vi "VI Tree.vi"   [LabVIEW 2018, in "TCPServer.lvlib"]
uses:
  TCPServer.lvlib
  TypeDefs/Sec Hdr CMD.ctl
  TypeDefs/Sec Hdr TLM.ctl
  TypeDefs/Connection.ctl
  TypeDefs/App.ctl
  TypeDefs/CCSDS.ctl
  fd051608-15b4-44f6-a0b0-4995f7a393de.vi
types:
  T1 = typedef "TCPServer.lvlib/Connection.ctl" = cluster{"Tcp":refnum<k5>, "Server Port":u16, "Server Port Type":enum8{"CMD", "TLM", "BOTH"}, "Client IP":string, "Client Port":u16}
  T2 = typedef "TCPServer.lvlib/CCSDS.ctl" = cluster{"Version":u8, "Type":enum8{"TLM", "CMD"}, "SecHdrFlag":bool, "AppID":u16, "SeqFlags":u8, "SeqCount":u16, "PktLength":u16}
  T3 = typedef "TCPServer.lvlib/App.ctl" = cluster{"Stack":refnum<queue>, "Cmd":cluster{"Conn":refnum<data-value>, "Daemon":refnum<vi>, "Counter":refnum<data-value>}, "Tlm":cluster{"Conn":refnum<data-value>, "Daemon":refnum<vi>, "Counter":refnum<data-value>}}
  T4 = typedef "TCPServer.lvlib/Sec Hdr TLM.ctl" = cluster{"DAYS_SINCE_2000":u16, "SECONDS_SINCE_START":u32, "MS_SINCE_START":u16}
  T5 = typedef "TCPServer.lvlib/Sec Hdr CMD.ctl" = cluster{"CMD_ID":u8, "CMD_CHECKSUM":u8}
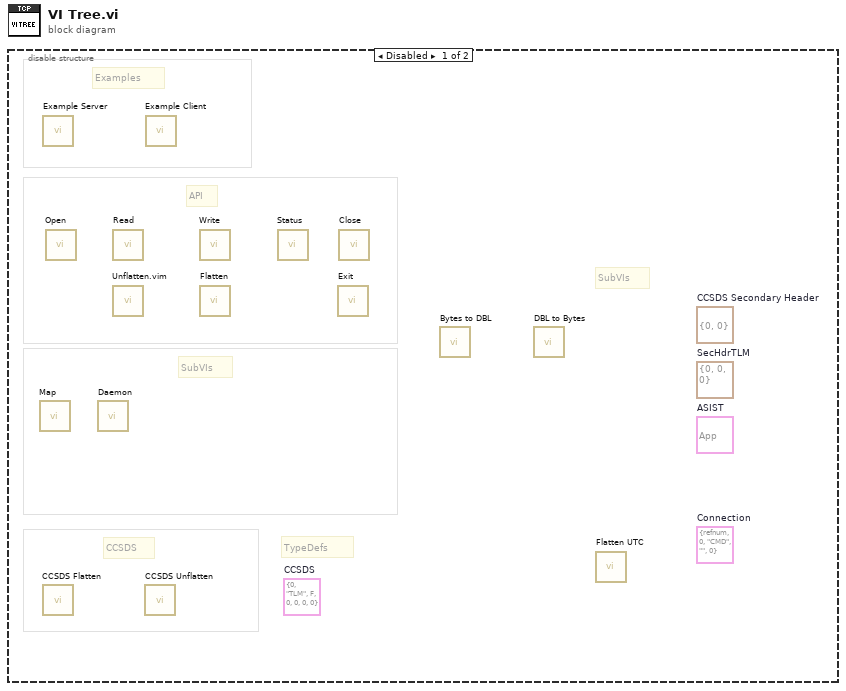
[diagram p0: block diagram]
diagram:
  n1 = disable-structure shown="Disabled" {
    frame Disabled {
      (unwired) T1 {"Tcp"=refnum, "Server Port"=0, "Server Port Type"=enum."CMD", "Client IP"="", "Client Port"=0}  # Connection
      (unwired) T2 {"Version"=0, "Type"=enum."TLM", "SecHdrFlag"=FALSE, "AppID"=0, "SeqFlags"=0, "SeqCount"=0, "PktLength"=0}  # CCSDS
      (unwired) T3 {"Stack"=refnum, "Cmd"={"Conn"=refnum, "Daemon"=refnum, "Counter"=refnum}, "Tlm"={"Conn"=refnum, "Daemon"=refnum, "Counter"=refnum}}  # ASIST
      (unwired) T4 {"DAYS_SINCE_2000"=0, "SECONDS_SINCE_START"=0, "MS_SINCE_START"=0}  # SecHdrTLM
      (unwired) T5 {"CMD_ID"=0, "CMD_CHECKSUM"=0}  # CCSDS Secondary Header
      # "CCSDS"
      # "SubVIs"
      # "API"
      # "TypeDefs"
      # "SubVIs"
      # "Examples"
      n2 = call "Map.vi"() -> ()  [unwired: 9 in, 3 out]
      n3 = call "Example Server.vi"() -> ()  [unwired: 12 in]
      n4 = call "CCSDS Flatten.vi"() -> ()  [unwired: 10 in, 2 out]
      n5 = call "Open.vi"() -> ()  [unwired: 9 in, 3 out]
      n6 = call "Daemon.vi"() -> ()  [unwired: 12 in]
      n7 = call "Read.vi"() -> ()  [unwired: 7 in, 5 out]
      n8 = call "Unflatten.vim"() -> ()  [unwired: 9 in, 3 out]
      n9 = call "CCSDS Unflatten.vi"() -> ()  [unwired: 9 in, 3 out]
      n10 = call "Example Client.vi"() -> ()  [unwired: 12 in]
      n11 = call "Write.vi"() -> ()  [unwired: 10 in, 2 out]
      n12 = call "Flatten.vi"() -> ()  [unwired: 10 in, 2 out]
      n13 = call "Status.vi"() -> ()  [unwired: 5 in, 7 out]
      n14 = call "Exit.vi"() -> ()  [unwired: 10 in, 2 out]
      n15 = call "Close.vi"() -> ()  [unwired: 11 in, 1 out]
      n16 = call "Bytes to DBL.vi"() -> ()  [unwired: 11 in, 1 out]
      n17 = call "DBL to Bytes.vi"() -> ()  [unwired: 11 in, 1 out]
      n18 = call "Flatten UTC.vi"() -> ()  [unwired: 11 in, 1 out]
    }
    frame Enabled {
    }
  }
